vi "find the max-min.vi"() -> ()   [LabVIEW 2018]
uses:
  <vilib>/Utility/file.llb/Read Delimited Spreadsheet (DBL).vi
panel:
  out "Prepared by \nthe project":string
  out "Min":dbl
  out "Max":dbl
  out "Daata":dbl[][](array[numeric])
  in  "Measurement file \nwith extension Txt":path
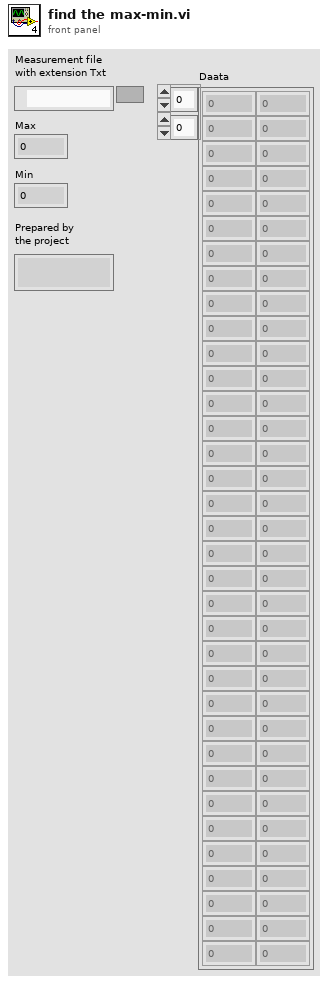
[diagram p1: front panel]
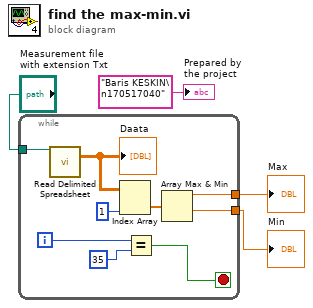
[diagram p0: block diagram]
diagram:
  n1 = while {
    tunnel: "Measurement file \nwith extension Txt" -> [w13]
    tunnel: [w6] -> w3
    tunnel: [w5] -> w2
    i -> [w9]
    stop <- w8 stop-if-true
    n2 = call-poly <vilib>:"Read Delimited Spreadsheet.vi"("file path (dialog if empty)"=w13) -> ("all rows"=w10:dbl[][])  [unwired: 9 in, 5 out]
    "Daata" <- w10
    n3 = Index Array(array=w10, index (col)=1 ("disabled index (col)")) -> (element=w11:dbl[])  [unwired: 1 in]
    n4 = Equal?(x=w9, y=35) -> (x = y?=w8:bool)
    n5 = Array Max & Min(array=w11) -> (max value=w6:dbl, min value=w5:dbl)  [unwired: 2 out]
  }
  "Max" <- w3
  "Min" <- w2
  "Prepared by \nthe project" <- "Baris KESKIN\n170517040"
